vi "snapImgFULL.vi"(1 "Index":i32, 2 "filename":string="testImg", 3 "Base path":path=path "C:/Users/sims01/Desktop/dataAcq", 4 "sCMOS cluster":cluster{"init":i16, "sCMOS handle":u32}) -> (0 "Full file":path=path "C:/Users/LSFM_2/Desktop/dataAcq_2705/bothIllAxis/4umBead0.tif")   [LabVIEW 2015]
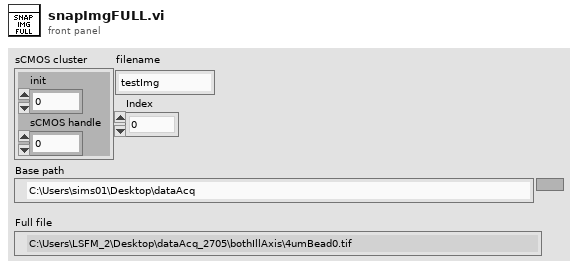
[diagram p1: front panel]
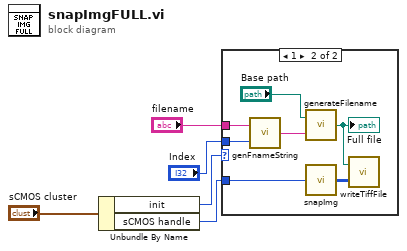
[diagram p0: block diagram]
diagram:
  n1 = Unbundle By Name("sCMOS cluster") -> ("init"=w4:i16, "sCMOS handle"=w1:u32)
  n2 = case shown="1" w4 {
    tunnel: "filename" -> [_ w12]
    tunnel: "Index" -> [_ w11]
    tunnel: w1 -> [_ w10]
    frame 0, Default {
    }
    frame 1 {
      n3 = call "genFnameString.vi"("Idx"=w11, "str"=w12) -> ("fName"=w8:string)
      n4 = call "generateFilename.vi"("Filename"=w8, "Base path"="Base path") -> ("Appended path"=w6:path)
      "Full file" <- w6
      n5 = call "snapImg.vi"("Handle in"=w10) -> ("16bitImgFile"=w9:u16[][])
      n6 = call "writeTiffFile.vi"("Image Pixels (U16)"=w9, "File Path"=w6) -> ()
    }
  }
